vi "DSF.Engine.BuilderManager.Pool.Return Builder.vi"(8 "error in (no error)":errorcluster, 9 "timeout in ms":i32 format="%d ms", 10 "Builder":refnum<class "DSF.Engine.Builder.lvclass">, 11 "Builder Manager in":refnum<class "DSF.Engine.BuilderManager.lvclass">) -> (0 "error out":errorcluster, 1 "timed out?":bool, 3 "Builder Manager out":refnum<class "DSF.Engine.BuilderManager.lvclass">)   [LabVIEW 2016, in "DSF.Engine.lvlib" / "DSF.Engine.BuilderManager.lvclass"]
uses:
  DSF.Engine.BuilderManager.lvclass
  Builder/DSF.Engine.Builder.lvclass
  Builder/DSF.Engine.Builder.lvclass/DSF.Engine.Builder.ctl
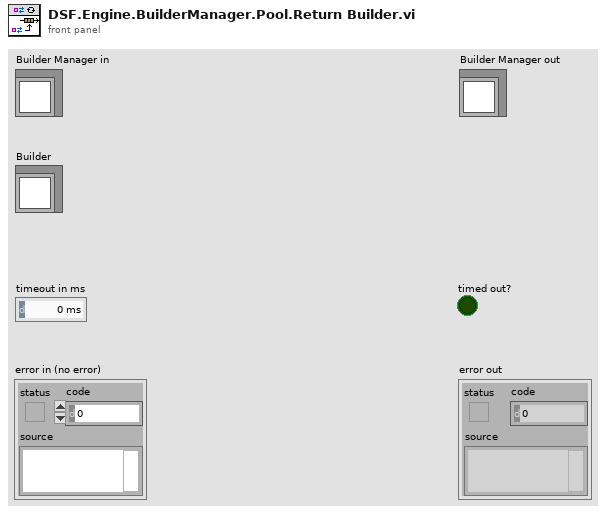
[diagram p1: front panel]
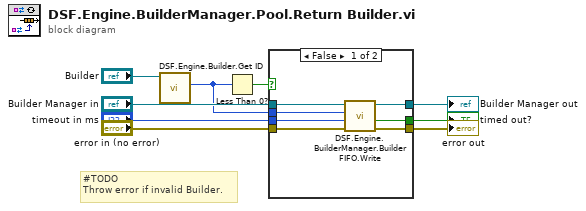
[diagram p0: block diagram]
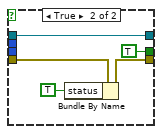
[diagram p2: hidden frame]
diagram:
  # "#TODO\nThrow error if invalid Builder."
  n1 = call "DSF.Engine.Builder.Get ID.vi"("Builder in"="Builder") -> ("ID"=w3:i32)  [unwired: 9 in, 1 out]
  n2 = Less Than 0?(x=w3) -> (x < 0?=w4:bool)
  n3 = case shown="False" w4 {
    tunnel: "Builder Manager in" -> [w16 w21]
    tunnel: "error in (no error)" -> [w15 w20]
    tunnel: [w14 w19] -> w7
    tunnel: [w13 w21] -> w6
    tunnel: w3 -> [w12 _]
    tunnel: "timeout in ms" -> [w11 _]
    tunnel: [w10 TRUE ("timed out?")] -> w1
    frame False {
      n4 = call "DSF.Engine.BuilderManager.Builder FIFO.Write.vi"("error in (no error)"=w15, "timeout in ms (0)"=w11, "Builder ID"=w12, "Builder Manager in"=w16) -> ("error out"=w14:errorcluster, "timed out?"=w10:bool, "Builder Manager out"=w13:refnum<class "DSF.Engine.BuilderManager.lvclass">)  [unwired: 5 in]
    }
    frame True {
      n5 = Bundle By Name(cluster=w20, "status"=TRUE) -> (w19:errorcluster)
    }
  }
  "error out" <- w7
  "Builder Manager out" <- w6
  "timed out?" <- w1
